vi "Translator.File.Find.vi"(8 "error in":errorcluster, 11 "Translation folder":path=path "D:/PL_0125_Sapphire_Automation/settings") -> (0 "error out":errorcluster, 2 "Languages":string[](array[string]))   [LabVIEW 2016]
uses:
  Translator.Enums.ctl
  Translator.Message.ctl
  EventLog/EventLog.EventLevelGui.ctl
  Windows/Windows.ExitAction.ctl
  TouchPanel/TouchPanelMonths.ctl
  EventLog/EventLog.EventSource.ctl
panel:
  in  "Enums":T1={"Msg"=enum."Quitting", "Level"=enum."ALL", "ExitAction"=enum."Log off from PC", "Month"=enum."January", "Source"=enum."Gui"}
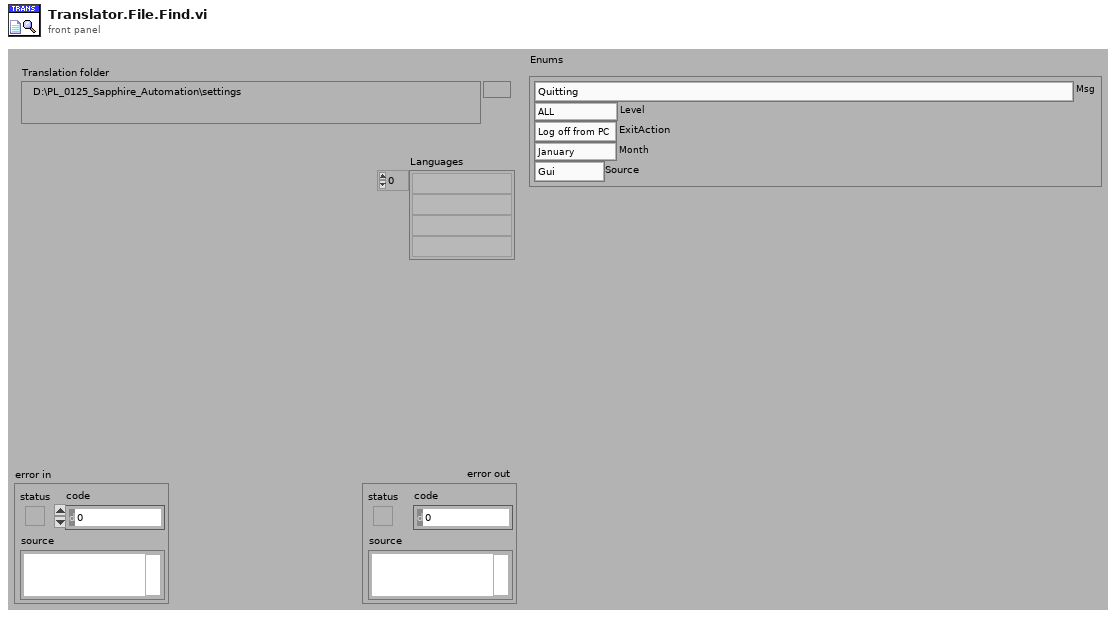
[diagram p1: front panel]
types:
  T1 = typedef "Translator.Enums.ctl" = cluster{"Msg":T2, "Level":T3, "ExitAction":T4, "Month":T5, "Source":T6}
  T2 = typedef "Translator.Message.ctl" = enum16{"-", "Event confirmed", "Log out", "Log in", "Shutdown", "Cancel", "Start", "Continue", "Stop", "On", "Off", "OK", "NOK", "NOK %s", "This", "Prev", "Home", "Work", "In progress...", "Missing", "Empty", "Hardware failure", "Initial", "Error %d >> %s", "Error %d >> %s >> %s", "Starting %s", "Quitting %s", "Configured", "Initializing", "Quitting", "Loading", "Running %s", "Stopped", "Summary", "Do you want to continue?", "Do you want to exit?", "Log out?", "System", "All", "IDLE", "Translating...%s", "Not found", "Alarm %s", "Run", "Skip", "Abort", "Repeat", "Please wait...", "Database disconnected", "Login to database successful", "Login to database failed: %d; %s", "Get process step data for %s", "Changeover off", "Changeover into %s", "Product %s | %s found in cache with status %d at previous station", "Product %s | %s found in database with status %d at previous station", "Product %s | %s not found in cache at previous station", "Product %s | %s not found in database at previous station", "Product %s | %s found in cache with status %d at this station (%d repetion)", "Product %s | %s found in database with status %d at this station (%d repetition)", "Product %s | %s not found in cache at this station", "Product %s | %s not found in database at this station", "Product %s | %s found in cache for component %s | %s", "Product %s | %s found in database for component %s | %s", "Product not found in cache for component %s | %s", "Product not found in database for component %s | %s", "Product %s | %s connected with component %s | %s (cache)", "Product %s | %s connected with component %s | %s (database)", "New data for %s | %s (cache)", "New data for %s | %s (database)", "File %s moved (cache)", "File %s deleted (cache)", "Msg %d >> %s", "PLC LifeBit Failure", "Reconnecting DB", "Reconnecting PLC", "Free disk space is below 1GB - contact technician", "Unable to check product status"}
  T3 = typedef "EventLog.EventLevelGui.ctl" = enum16{"ALL", "Debug", "Info", "Warning", "Error"}
  T4 = typedef "Windows.ExitAction.ctl" = enum16{"Log off from PC", "Shut Down PC", "Reboot PC", "Close Program"}
  T5 = typedef "TouchPanelMonths.ctl" = enum16{"January", "February", "March", "April", "May", "June", "July", "August", "September", "October", "November", "December"}
  T6 = typedef "EventLog.EventSource.ctl" = enum16{"All", "Gui", "Cache", "PLC1", "PLC2", "PLC3", "DB", "DB01", "DB02", "DB03", "DB04", "DB05", "DB06", "DB07", "DB08", "DB09", "DB10", "DB11", "DB12", "DB13", "DB14", "DB15", "DB16"}
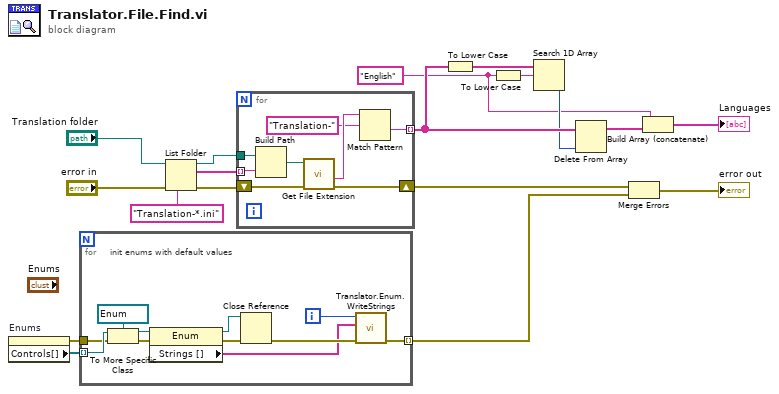
[diagram p0: block diagram]
diagram:
  w5 = "English" ("element")
  n1 = property on="Enums" class="Clust (strict)"() -> (error out=w3:errorcluster, "Controls[]"=w4:refnum<vi>[])  [unwired: 2 in, 1 out]
  n2 = for {
    tunnel: w4 -> [w29] mode=indexing
    tunnel: w3 -> [w26]
    tunnel: [w23] -> w1 mode=indexing
    i -> [w20]
    # "init enums with default values"
    n3 = To More Specific Class(target class=refnum<vi> refnum ("reference out"), reference=w29, error in=w26) -> (specific class reference=w19:refnum<vi>, error out=w28:errorcluster)
    n4 = property class="Enum"(reference=w19, error in=w28) -> (reference out=w24:refnum<vi>, error out=w25:errorcluster, "Strings []"=w21:string[])
    n5 = Close Reference(reference=w24, error in (no error)=w25) -> (error out=w22:errorcluster)
    n6 = call "Translator.Enum.WriteStrings.vi"("error out"=w22, "Strings"=w21, "idx"=w20) -> ("error out 2"=w23:errorcluster)  [unwired: 8 in]
  }
  n7 = List Folder(path="Translation folder", pattern="Translation-*.ini", error in="error in") -> (path out=w11:path, filenames=w12:string[], error out=w13:errorcluster)  [unwired: 1 in, 1 out]
  n8 = for {
    tunnel: w12 -> [w36] mode=indexing
    tunnel: w11 -> [w37]
    tunnel: [w30] -> w9 mode=indexing
    shift-right: [w33] -> w17
    shift-left: w13 -> [w34]
    n9 = Build Path(base path=w37, name or relative path=w36) -> (appended path=w35:path)
    n10 = call <vilib>:"Get File Extension.vi"("error in (no error)"=w34, "file"=w35) -> ("error out"=w33:errorcluster, "filename without extension"=w32:string)  [unwired: 5 in, 3 out]
    n11 = Match Pattern(string=w32, regular expression="Translation-" ("pattern")) -> (after substring=w30:string)  [unwired: 1 in, 3 out]
  }
  n12 = To Lower Case(string=w9) -> (all lower case string=w10:string[])
  n13 = To Lower Case(string=w5) -> (all lower case string=w6:string)
  n14 = Search 1D Array(1D array=w10, element=w6) -> (index of element=w7:i32)  [unwired: 1 in]
  n15 = Delete From Array(array=w9, index=w7) -> (array with subset deleted=w8:string[])  [unwired: 1 in, 1 out]
  n16 = Merge Errors(w17, w1) -> (→"error out":errorcluster)
  n17 = Build Array (concatenate)(w5, w8) -> (→"Languages":string[])
